vi "Wake HL.vi"(8 "error in (no error)":errorcluster, 10 "event data":T1={"Timeout"=0, "Instrument Channel"="", "Address"=0, "Current state"=enum."Configuration", "Desired state"=enum."Configuration", "Module ID"=0}, 11 "event cluster":T3) -> (0 "error out":errorcluster)   [LabVIEW 2020, in "FCR100.lvlib"]
uses:
  FCR100.lvlib
  Wake HL data -- cluster.ctl
  Device state -- enum.ctl
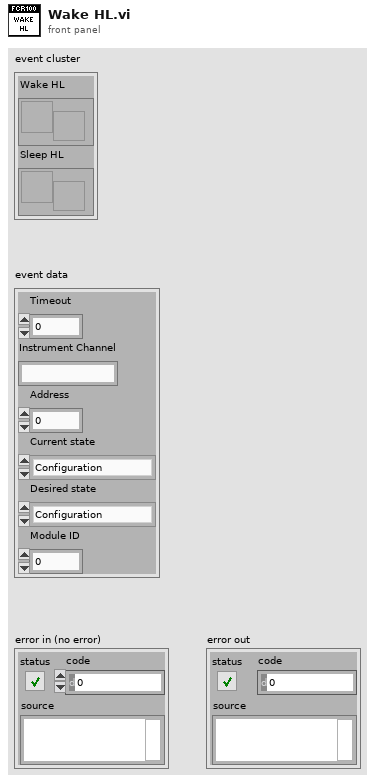
[diagram p1: front panel]
types:
  T1 = typedef "FCR100.lvlib/Wake HL data -- cluster.ctl" = cluster{"Timeout":i32, "Instrument Channel":string, "Address":u8, "Current state":T2, "Desired state":T2, "Module ID":i32}
  T2 = typedef "FCR100.lvlib/Device state -- enum.ctl" = enum16{"Not referenced", "Configuration", "Disable", "Ready", "Homing", "Motion"}
  T3 = cluster{"Wake HL":refnum<user-event>, "Sleep HL":refnum<user-event>}
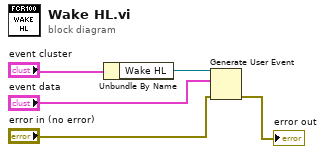
[diagram p0: block diagram]
diagram:
  n1 = Unbundle By Name("event cluster") -> ("Wake HL"=w2:refnum<user-event>)
  n2 = Generate User Event(user event=w2, event data cluster="event data", error in="error in (no error)") -> (error out=→"error out":errorcluster)  [unwired: 1 in, 1 out]
